vi "hmp4000 Configure Current Value.vi"(8 "error in (no error)":errorcluster, 9 "Current (0.0)":dbl format="%.3f", 11 "VISA resource name":refnum<visa-resource-name>) -> (0 "error out":errorcluster, 3 "VISA resource name out":refnum<visa-resource-name>)   [LabVIEW 2022 SP3]
doc: "This VI adjusts the output current.\n\nAttribute:\nHMP4000_ATTR_OUTPUT_CURRENT_LEVEL\n\nRemote-control command:\nSOURce:CURRent:LEVel:AMPLitude"
uses:
  Instance           1 39Saved   hmp4000 Configure Current Value .vi
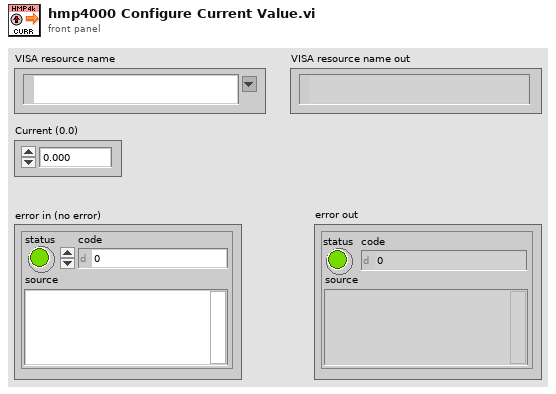
[diagram p1: front panel]
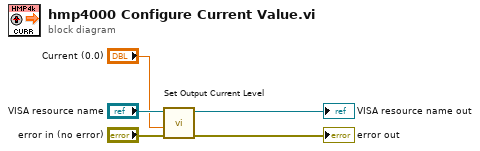
[diagram p0: block diagram]
diagram:
  n1 = call "Set Output Current Level"("error in (no error)"="error in (no error)", "Output Current Level (0.0)"="Current (0.0)", "instrument handle"="VISA resource name") -> ("error out"=→"error out":errorcluster, "instrument handle out"=→"VISA resource name out":refnum<visa-resource-name>)  [unwired: 7 in]
